vi "Test Instrument App.vi"() -> (0 "error out":errorcluster, 2 "loop":i32, 3 "pkg recived":timestamp)   [LabVIEW 2019]
uses:
  <vilib>/addons/zeromq/socket_type.ctl
  <vilib>/Field R&D Services/Logger/Type Definitions/Configuration.ctl
  <vilib>/Field R&D Services/Logger/Type Definitions/Severity.ctl
  mmWave_driver_Py/LV-API/mmW_commands/TypeDefs/response status.ctl
  mmWave_driver_Py/LV-API/mmW_commands/TypeDefs/commands.ctl
  <vilib>/Field R&D Services/Logger/Support/Create Level String.vi
  <vilib>/Field R&D Services/Logger/Support/Strip Whitespace.vi
  <vilib>/dlg_ctls.llb/Space Constant.vi
  <vilib>/Field R&D Services/Logger/Support/Manager.vi
  <vilib>/Utility/error.llb/Trim Whitespace.vi
  <vilib>/Field R&D Services/Logger/Support/Control State.vi
  <vilib>/addons/zeromq/zmq_context.lvclass
  <vilib>/addons/zeromq/zmq_socket.lvclass
  <vilib>/addons/zeromq/zeromq.lvlib
  <vilib>/Field R&D Services/Logger/Field_RnD_Services_Logger_Toolkit.lvlib
  mmWave_driver_Py/LV-API/mmW_commands/mmW_commands.lvlib
  Service.lvlib
panel:
  in  "Tab Control":enum32{"Messages", "Settings", "Debug"}(tab)
  out "parts":string[](array[string])
  out "Mode":enum16{"RF", "IF", "BB"}(ring)
  out "2D-IQ":dbl[][](graph)
  in  "Log Root Folder":path
  in  "ZMQ Server":string="tcp://127.0.0.1:5555"
  out "Messages":i32(listbox)
  in  "stop":bool
  # "Test Instrument Application"
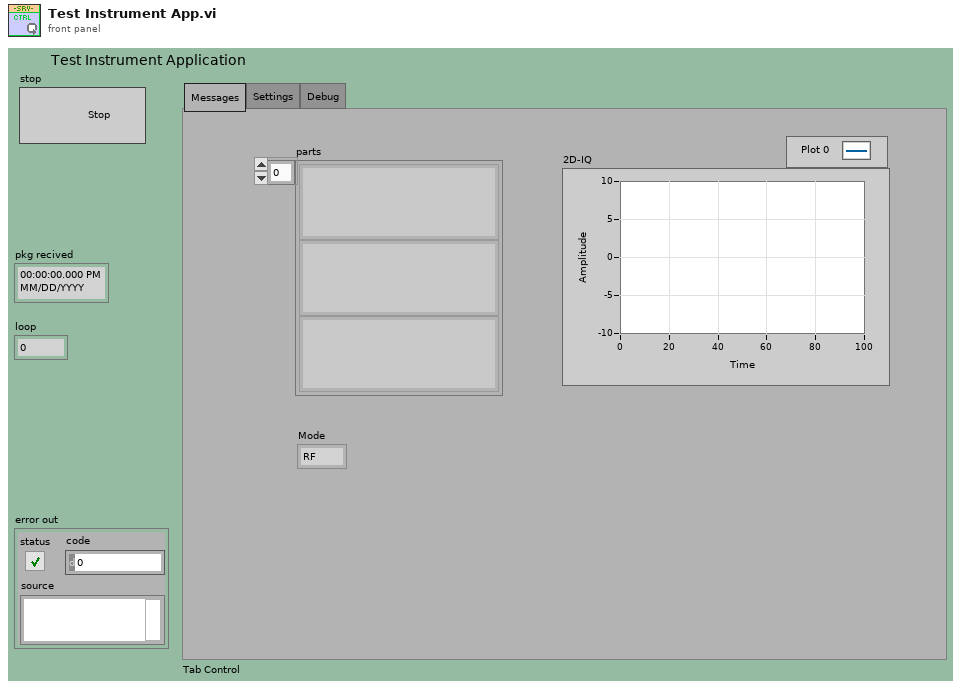
[diagram p1: front panel]
types:
  T1 = typedef "Field_RnD_Services_Logger_Toolkit.lvlib/Severity.ctl" = enum16{"Benign", "Warning", "Recoverable", "Fatal"}
  T2 = typedef "Field_RnD_Services_Logger_Toolkit.lvlib/Configuration.ctl" = cluster{"Delimiter":string, "Enable Calendar Tree":bool, "File Extension":string, "Maximum File Count":i32, "Maximum File Size":i64, "Prune All":bool, "Root Folder":path}
  T3 = typedef "zeromq.lvlib/socket_type.ctl" = enum8{"ZMQ_PAIR", "ZMQ_PUB", "ZMQ_SUB", "ZMQ_REQ", "ZMQ_REP", "ZMQ_DEALER", "ZMQ_ROUTER", "ZMQ_PULL", "ZMQ_PUSH", "ZMQ_XPUB", "ZMQ_XSUB"}
  T4 = typedef "mmW_commands.lvlib/commands.ctl" = enum16{"configure_fs", "configure_rf", "configure_trigger", "equalization_enable", "equalization_start", "lo_sync_enable", "equalization_stop", "get_instrument_status", "get_versions", "initialize_hw", "pop_rx", "set_log_level", "Shutdown", "start", "start_instrument_app", "stop", "transceive", "trigger_burst", "trigger_sync_enable", "Write TX", "resp_generic", "resp_waveform"}
  T5 = typedef "mmW_commands.lvlib/response status.ctl" = enum16{"OK", "Error", "Warning", "Unknown"}
  T6 = typedef "mmW_commands.lvlib/command_types.ctl" = enum16{"invalid_command", "instrument_control", "environment_control", "response"}
  T7 = typedef "mmW_commands.lvlib/mode.ctl" = enum16{"RF", "IF", "BB"}
  T8 = typedef "Logger.lvlib/Statement.ctl" = cluster{"Time Stamp":timestamp, "Tag":T9, "Source":string, "Message":string}
  T9 = typedef "Logger.lvlib/Tag.ctl" = enum16{"Fatal", "Error", "Warn", "Info", "Debug", "Trace"}
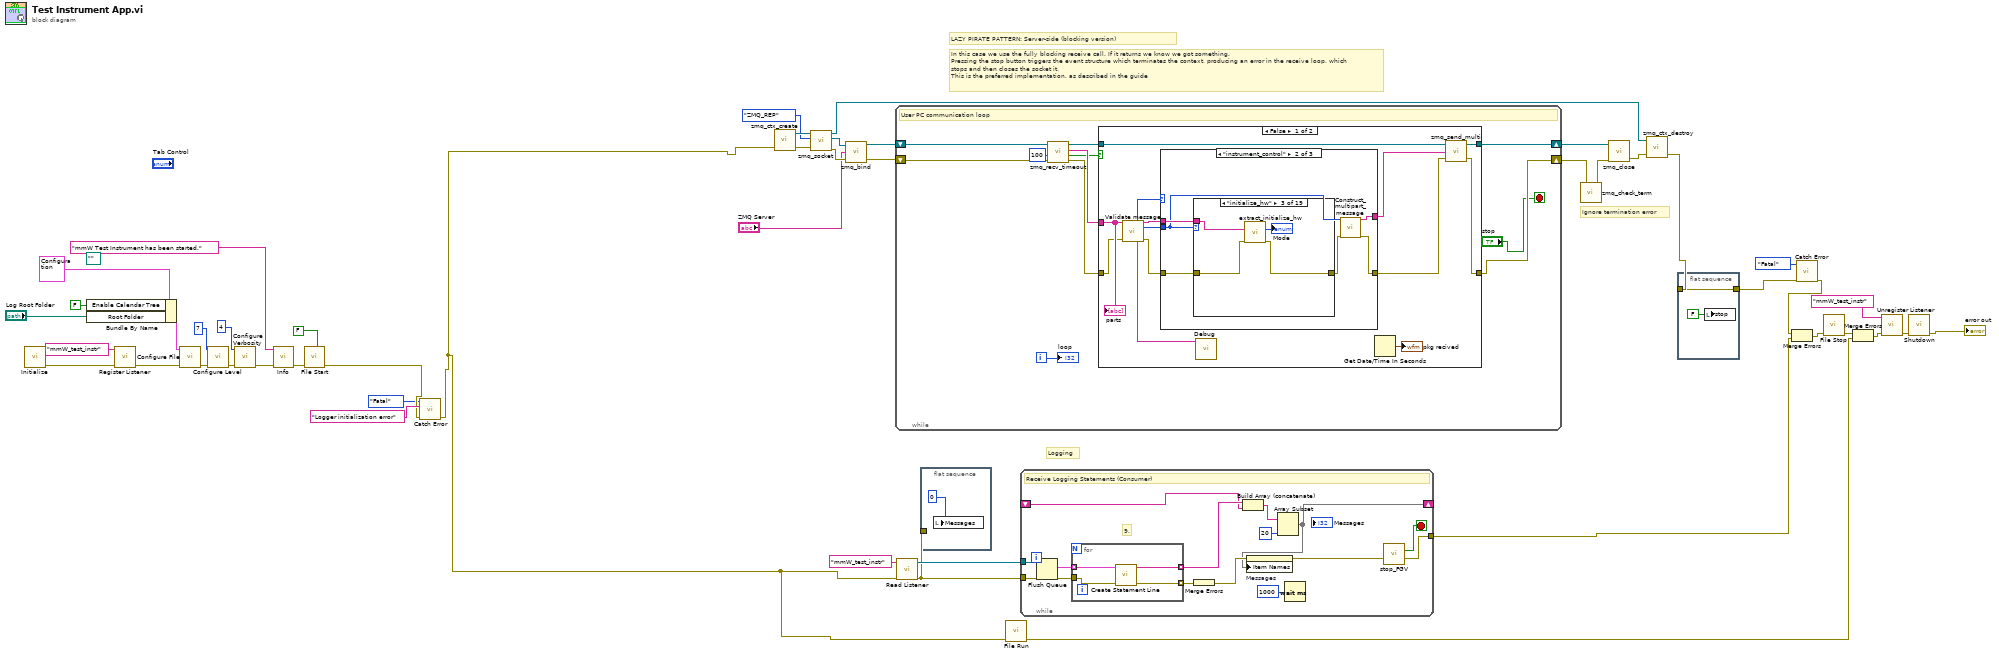
[diagram p0: block diagram]
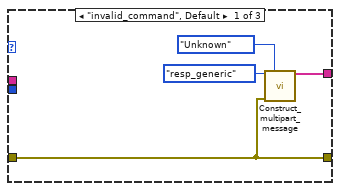
[diagram p2: hidden frame]
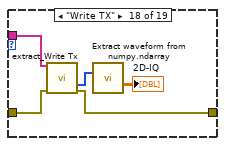
[diagram p19: hidden frame]
diagram:
  (unwired) path "" ("Log files path")
  # "Logging"
  # "In this case we use the fully blocking receive call. If it returns we know we got something.\nPressing the stop button triggers the event structure which terminates the context, producing an error in the receive loop, which stops and then closes the socket it.\nThis is the preferred implementation, as described in the guide"
  # "LAZY PIRATE PATTERN: Server-side (blocking version)"
  # "Ignore termination error"
  n1 = call <vilib>:"Initialize.vi"() -> ("Error Out"=w16:errorcluster)  [unwired: 11 in]
  n2 = Bundle By Name(cluster=T2 {"Delimiter"=",", "Enable Calendar Tree"=TRUE, "File Extension"="csv", "Maximum File Count"=5, "Maximum File Size"=15728640, "Prune All"=FALSE, "Root Folder"=path ""} ("Configuration"), "Enable Calendar Tree"=FALSE, "Root Folder"="Log Root Folder") -> (w15:T2)
  n3 = call <vilib>:"Register Listener.vi"("Error In"=w16, "Listener ID"="mmW_test_instr") -> ("Error Out"=w17:errorcluster)  [unwired: 9 in]
  n4 = call <vilib>:"Configure File.vi"("Error In"=w17, "Configuration"=w15) -> ("Error Out"=w19:errorcluster)  [unwired: 9 in]
  n5 = call <vilib>:"Configure Level.vi"("Error In"=w19, "Level"=u8 7) -> ("Error Out"=w20:errorcluster)  [unwired: 9 in]
  n6 = call <vilib>:"Configure Verbosity.vi"("Error In"=w20, "Verbosity"=u8 4) -> ("Error Out"=w23:errorcluster)  [unwired: 9 in]
  n7 = call <vilib>:"Info.vi"("Error In"=w23, "Message"="mmW Test Instrument has been started.") -> ("Error Out"=w24:errorcluster)  [unwired: 9 in]
  n8 = call <vilib>:"File Start.vi"("Run in Background"=FALSE, "Error In"=w24) -> ("Error Out"=w27:errorcluster)  [unwired: 9 in]
  n9 = call <vilib>:"Catch Error.vi"("Error In"=w27, "Source"="Logger initialization error", "Severity"=Severity."Fatal") -> ("Error Out"=w11:errorcluster)  [unwired: 8 in]
  n10 = call <vilib>:"zmq_ctx_create.vi"("error in"=w11) -> ("error out"=w42:errorcluster, "context out"=w38:refnum<class "zmq_context.lvclass">)  [unwired: 3 in]
  n11 = call <vilib>:"zmq_socket.vi"("error in"=w42, "socket type"=socket_type."ZMQ_REP", "context in"=w38) -> ("error out"=w43:errorcluster, "socket out"=w39:refnum<class "zmq_socket.lvclass">, "context out"=w45:refnum<class "zmq_context.lvclass">)  [unwired: 2 in]
  n12 = call <vilib>:"zmq_bind.vi"("error in"=w43, "endpoint"="ZMQ Server", "socket in"=w39) -> ("error out"=w44:errorcluster, "socket out"=w35:refnum<class "zmq_socket.lvclass">)  [unwired: 1 in]
  n13 = while {
    shift-right: [w50] -> w37
    shift-left: w35 -> [w58]
    shift-right: [w49] -> w40
    shift-left: w44 -> [w56]
    i -> [w57]
    stop <- "stop" stop-if-true
    # "User PC communication loop"
    n14 = call <vilib>:"zmq_recv_timeout.vi"("error in"=w56, "timeout (ms)"=u32 100, "socket in"=w58) -> ("error out"=w54:errorcluster, "timeout?"=w52:bool, "parts"=w55:string[], "socket out"=w51:refnum<class "zmq_socket.lvclass">)  [unwired: 1 in]
    n15 = case shown="False" w52 {
      tunnel: w55 -> [w66 _]
      tunnel: w54 -> [w65 w113]
      tunnel: [w67 w113] -> w49
      tunnel: w51 -> [w71 w112]
      tunnel: [w70 w112] -> w50
      frame False {
        n16 = call "Validate message.vi"("multipart message in"=w66, "error in (no error)"=w65) -> ("Command Type"=w64:T6, "multipart message out"=w61:string[], "command out"=w62:T4, "Debug info"=w59:string, "error out"=w63:errorcluster)  [unwired: 8 in, 1 out]
        n17 = case shown="\"instrument_control\"" w64 {
          tunnel: w63 -> [w73 w80 w109]
          tunnel: [w73 w77 w109] -> w68
          tunnel: w62 -> [_ w79 _]
          tunnel: w61 -> [_ w81 _]
          tunnel: [w72 w76 w108] -> w60
          frame "invalid_command", Default {
            n18 = call "Construct_multipart_message.vi"("command"=commands."resp_generic", "Status"=response_status."Unknown", "error in (no error)"=w73) -> ("Multipart message"=w72:string[])  [unwired: 9 in, 3 out]
          }
          frame "instrument_control" {
            n19 = case shown="\"initialize_hw\"" w79 {
              tunnel: w81 -> [_ _ w87 _ _ _ _ _ _ _ _ _ _ _ _ _ _ w104 _]
              tunnel: w80 -> [w82 w83 w86 w88 w89 w90 w91 w92 w93 w94 w95 w96 w97 w98 w99 w100 w101 w106 w107]
              tunnel: [w82 w83 w85 w88 w89 w90 w91 w92 w93 w94 w95 w96 w97 w98 w99 w100 w101 w105 w107] -> w78
              frame "configure_rf", Default {
              }
              frame "configure_trigger" {
              }
              frame "initialize_hw" {
                n20 = call "extract_initialize_hw.vi"("multipart message in"=w87, "error in (no error)"=w86) -> ("Mode"=→"Mode":T7, "error out"=w85:errorcluster)  [unwired: 9 in, 3 out]
              }
              frame "pop_rx" {
              }
              frame "lo_sync_enable" {
              }
              frame "equalization_stop" {
              }
              frame "start" {
              }
              frame "stop" {
              }
              frame "trigger_burst" {
              }
              frame "Shutdown" {
              }
              frame "transceive" {
              }
              frame "resp_generic" {
              }
              frame "resp_waveform" {
              }
              frame "equalization_enable" {
              }
              frame "equalization_start" {
              }
              frame "set_log_level" {
              }
              frame "trigger_sync_enable" {
              }
              frame "Write TX" {
                n21 = call "extract_Write Tx.vi"("multipart message in"=w104, "error in (no error)"=w106) -> ("interleaved I16 wfm"=w103:i16[], "error out"=w105:errorcluster)  [unwired: 8 in, 4 out]
                n22 = call "Extract waveform from numpy.ndarray.vi"("I16"=w103) -> ("2D-IQ"=→"2D-IQ":dbl[][])  [unwired: 12 in, 2 out]
              }
              frame "configure_fs" {
              }
            }
            n23 = call "Construct_multipart_message.vi"("command"=w79, "error in (no error)"=w78) -> ("Multipart message"=w76:string[], "error out"=w77:errorcluster)  [unwired: 10 in, 2 out]
          }
          frame "environment_control" {
            n24 = call "Construct_multipart_message.vi"("command"=commands."resp_generic", "Status"=response_status."Unknown", "error in (no error)"=w109) -> ("Multipart message"=w108:string[])  [unwired: 9 in, 3 out]
          }
        }
        n25 = call <vilib>:"Debug.vi"("Message"=w59) -> ()  [unwired: 10 in, 1 out]
        n26 = Get Date/Time In Seconds() -> (seconds since 1Jan1904=→"pkg recived":timestamp)
        n27 = call <vilib>:"zmq_send_multi.vi"("error in"=w68, "parts"=w60, "socket in"=w71) -> ("error out"=w67:errorcluster, "socket out"=w70:refnum<class "zmq_socket.lvclass">)  [unwired: 1 in]
        "parts" <- w66
      }
      frame True {
      }
    }
    "loop" <- w57
  }
  n28 = call <vilib>:"Read Listener.vi"("Error In"=w11, "Listener ID"="mmW_test_instr") -> ("Error Out"=w30:errorcluster, "Listener"=w32:refnum<queue>)  [unwired: 8 in]
  n29 = flat-sequence {
    tunnel: w30 -> [_]
    frame #0 {
      n30 = local write "Messages"(0 ("Messages")) -> ()
    }
  }
  n31 = call <vilib>:"File Run.vi"("Error In"=w11) -> ("Error Out"=w4:errorcluster)  [unwired: 10 in]
  n32 = while {
    tunnel: w32 -> [w129]
    tunnel: w30 -> [w128]
    tunnel: [w115] -> w3
    shift-right: [w118] -> _
    shift-left: _ -> [w121]
    stop <- w116 stop-if-true
    # "9."
    # "Receive Logging Statements (Consumer)"
    n33 = Flush Queue(queue=w129, error in (no error)=w128) -> (remaining elements=w127:T8[], error out=w126:errorcluster)  [unwired: 1 out]
    n34 = for {
      tunnel: w127 -> [w133] mode=indexing
      tunnel: w126 -> [w132]
      tunnel: [w131] -> w122 mode=indexing
      tunnel: [w130] -> w125 mode=indexing
      n35 = call <vilib>:"Create Statement Line.vi"("Error In"=w132, "Statement"=w133) -> ("Error Out"=w130:errorcluster, "Line"=w131:string)  [unwired: 8 in]
    }
    n36 = Merge Errors(w125) -> (w124:errorcluster)
    n37 = Build Array (concatenate)(w122, w121) -> (w120:string[])
    n38 = Array Subset(array=w120, length=20) -> (w118:string[])  [unwired: 1 in]
    n39 = property on="Messages" class="LstBox (strict)"(error in=w124, "Item Names"=w118) -> (error out=w117:errorcluster)  [unwired: 1 in, 1 out]
    n40 = Wait (ms)(milliseconds to wait=u32 1000) -> ()  [unwired: 1 out]
    n41 = call "stop_FGV"("error in (no error)"=w117) -> ("stop?"=w116:bool, "error out"=w115:errorcluster)  [unwired: 13 in]
  }
  n42 = call <vilib>:"zmq_check_term.vi"("error in"=w40) -> ("error out"=w41:errorcluster)  [unwired: 1 in, 1 out]
  n43 = call <vilib>:"zmq_close.vi"("error in"=w41, "socket"=w37) -> ("error out"=w46:errorcluster)  [unwired: 3 in]
  n44 = call <vilib>:"zmq_ctx_destroy.vi"("error in"=w46, "context in"=w45) -> ("error out"=w33:errorcluster)  [unwired: 3 in]
  n45 = flat-sequence {
    tunnel: w33 -> [w135]
    tunnel: [w135] -> w2
    frame #0 {
      n46 = local write "stop"(FALSE ("stop")) -> ()
    }
  }
  n47 = call <vilib>:"Catch Error.vi"("Error In"=w2, "Severity"=Severity."Fatal") -> ("Error Out"=w1:errorcluster)  [unwired: 9 in]
  n48 = Merge Errors(w1, w3) -> (w6:errorcluster)
  n49 = call <vilib>:"File Stop.vi"("Error In"=w6) -> ("Error Out"=w8:errorcluster)  [unwired: 10 in]
  n50 = Merge Errors(w8, w4) -> (w10:errorcluster)
  n51 = call <vilib>:"Unregister Listener.vi"("Error In"=w10, "Listener ID"="mmW_test_instr") -> ("Error Out"=w9:errorcluster)  [unwired: 9 in]
  n52 = call <vilib>:"Shutdown.vi"("Error In"=w9) -> ("Error Out"=→"error out":errorcluster)  [unwired: 10 in]
